vi "Create Config File.vi"(11 "XML File Path":path) -> (3 "XML File Path(duplicate)":path)   [LabVIEW 2024, in "MQTTClient.lvlib"]
doc: "<b>Note:</b> This VI was modified by the <b>Validate DQMH Module</b> tool to turn off automatic error handling."
uses:
  MQTTClient.lvlib
  Config--cluster.ctl
  <vilib>/Utility/xml.llb/Write to XML File(string).vi
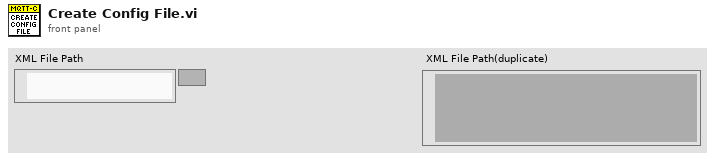
[diagram p1: front panel]
types:
  T1 = typedef "MQTTClient.lvlib/Config--cluster.ctl" = cluster{"Client-ID":string, "Server Address":string, "Server Port":u16}
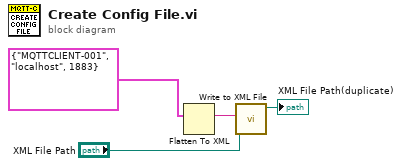
[diagram p0: block diagram]
diagram:
  n1 = Flatten To XML(6:T1 {"Client-ID"="MQTTCLIENT-001", "Server Address"="localhost", "Server Port"=1883} ("Configuration")) -> (2:w4:string)
  n2 = call-poly <vilib>:"Write to XML File.vi"("XML Input"=w4, "XML File Path"="XML File Path") -> ("XML File Path(duplicate)"=→"XML File Path(duplicate)":path)  [unwired: 7 in, 2 out]
